vi "Prediction.vi"(11 "Numeric":dbl) -> (3 "Numeric 2":dbl)   [LabVIEW 2017]
uses:
  <vilib>/Analysis/NI_AALPro.lvlib
panel:
  out "interpolation value":dbl format="%0.2f"
  in  "x value":dbl format="%0.2f"
  out "Waveform Chart":dbl(graph)
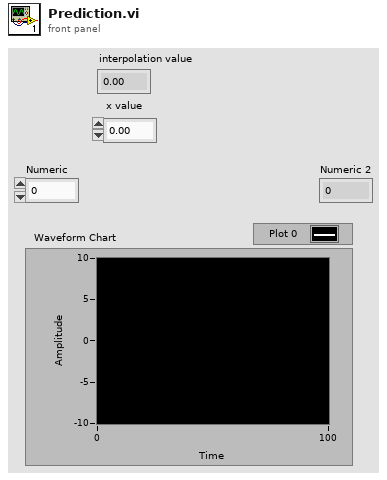
[diagram p1: front panel]
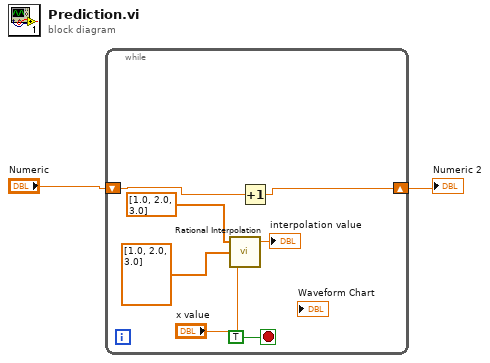
[diagram p0: block diagram]
diagram:
  n1 = while {
    shift-right: [w3] -> w1
    shift-left: "Numeric" -> [w4]
    stop <- TRUE stop-if-true
    n2 = call <vilib>:"Rational Interpolation.vi"("x value"="x value", "X"=dbl[] [1.0, 2.0, 3.0], "Y"=dbl[] [1.0, 2.0, 3.0]) -> ("interpolation value"=→"interpolation value":dbl)  [unwired: 2 out]
    n3 = Increment(x=w4) -> (x+1=w3:dbl)
  }
  "Numeric 2" <- w1
